vi "CAR Main.vi"(8 "error in (no error)":errorcluster) -> (0 "error out":errorcluster)   [LabVIEW 2009]
doc: "This is the main VI for the Cash Wash application. \nThis VI operates the touch-less car wash which is a car wash that relies on spray only, there are no brushes.\nSee Front Panel documentation for descriptions and tips on how to operate the car wash.\nSee Block Diagram documentation for more detailed information.\nThis VI uses a Producer Consumer (Events) Queued State Machine design pattern."
uses:
  controls/car_CarWashIndicators_cluster.ctl
  controls/car_CarWashSimulationSwitches_cluster.ctl
  controls/car_PurchaseSelection_cluster.ctl
  controls/car_ConsumerDataType_cluster.ctl
  controls/car_ConsumerCommand_enum.ctl
  modules/error/car_Error_Command_enum.ctl
  modules/car wash/car_CarWash_PurchaseSelection_enum.ctl
  modules/car wash/car_CarWash_Command_enum.ctl
panel:
  in  "Stop":bool
  in  "Simulation Switches":T1 caption="Car Wash Simulation Switches"
  out "Car Wash Indicators":T2
  in  "Purchase Selection":T3
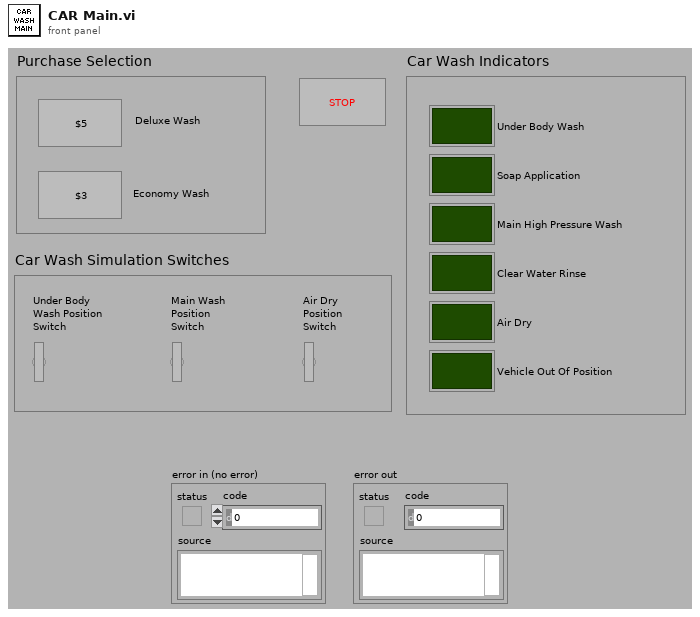
[diagram p1: front panel]
types:
  T1 = typedef "car_CarWashSimulationSwitches_cluster.ctl" = cluster{"Under Body Wash Position Switch":bool, "Main Wash Position Switch":bool, "Air Dry Position Switch":bool}
  T2 = typedef "car_CarWashIndicators_cluster.ctl" = cluster{"Under Body Wash":bool, "Soap Application":bool, "Main High Pressure Wash":bool, "Clear Water Rinse":bool, "Air Dry":bool, "Vehicle Out Of Position":bool}
  T3 = typedef "car_PurchaseSelection_cluster.ctl" = cluster{"Deluxe Wash":bool, "Economy Wash":bool}
  T4 = typedef "car_Error_Command_enum.ctl" = enum16{"Initialise", "Check for Error", "Report Errors"}
  T5 = typedef "car_ConsumerDataType_cluster.ctl" = cluster{"Command":T6, "Data":variant}
  T6 = typedef "car_ConsumerCommand_enum.ctl" = enum16{"Initialise", "Update Start Car Wash Display", "Start Wash", "Check Car Wash", "Car Wash Completed", "Exit"}
  T7 = typedef "car_CarWash_Command_enum.ctl" = enum16{"Initialise", "Start Car Wash", "Check Car Wash Cycle", "Next Cycle", "Shutdown"}
  T8 = enum8{"Enabled", "Disabled", "Disabled and Grayed Out"}
  T9 = typedef "car_CarWash_PurchaseSelection_enum.ctl" = enum16{"Economy", "Deluxe"}
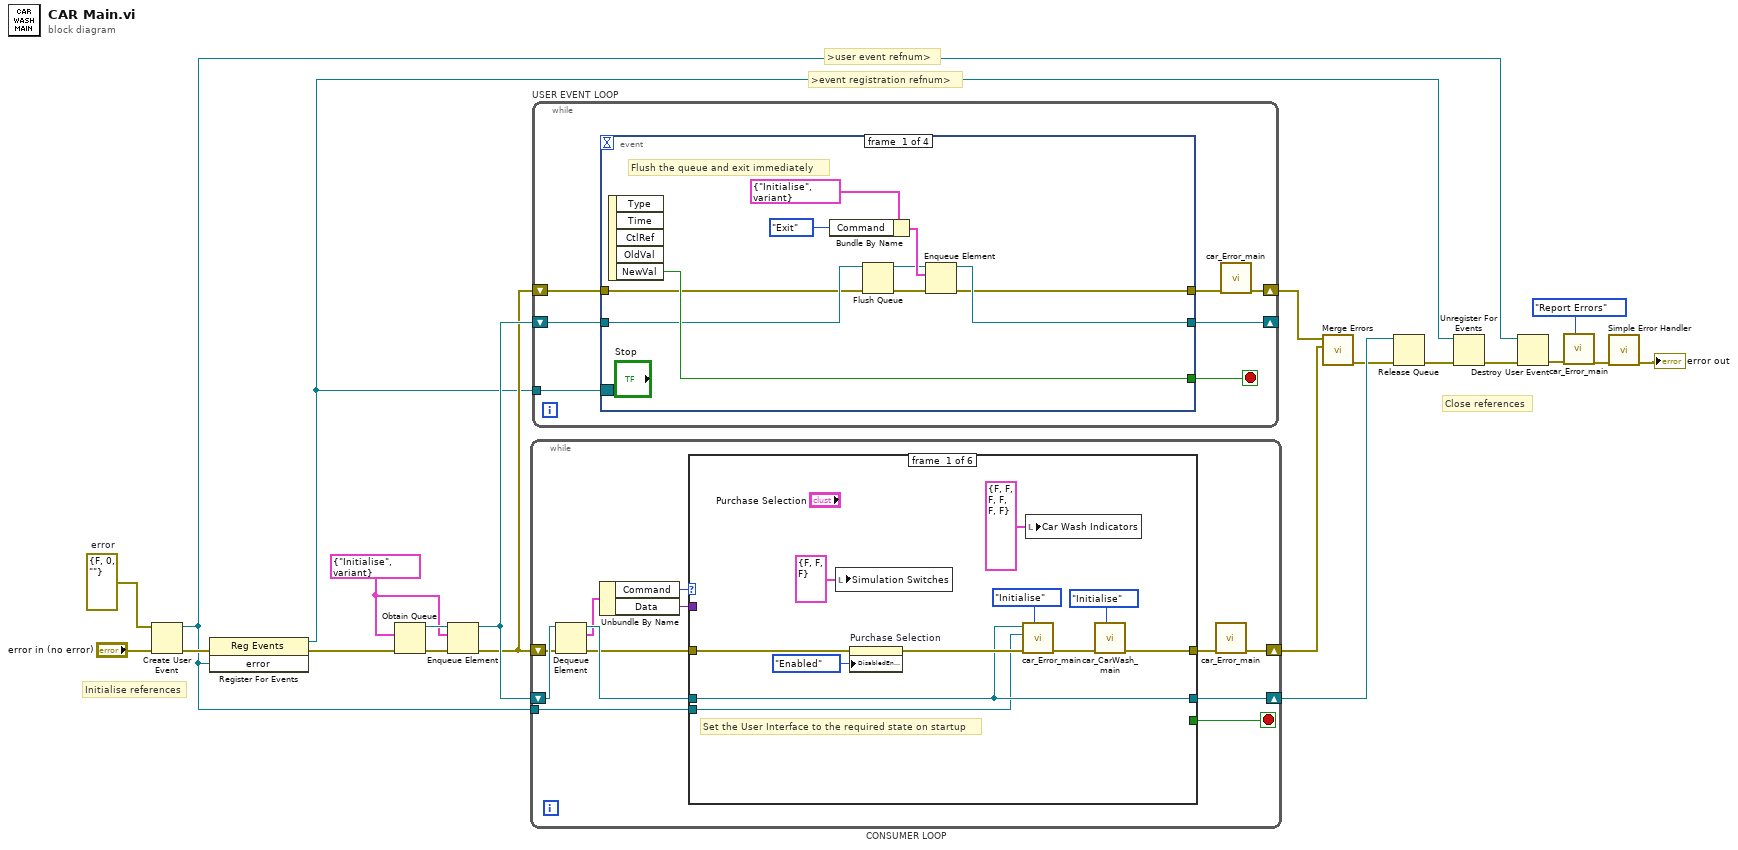
[diagram p0: block diagram]
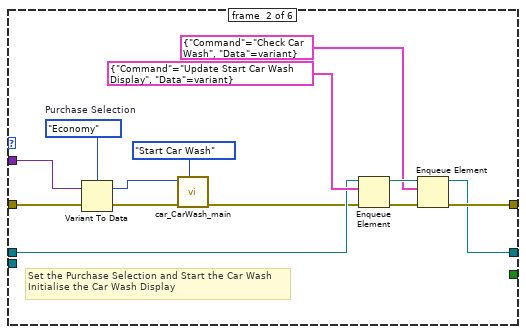
[diagram p2: hidden frame]
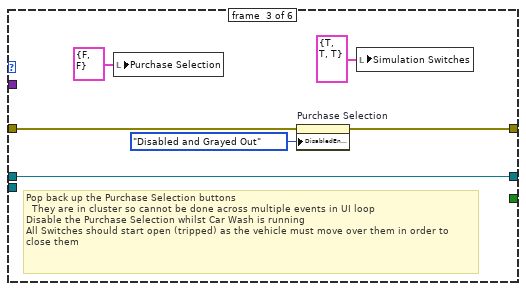
[diagram p3: hidden frame]
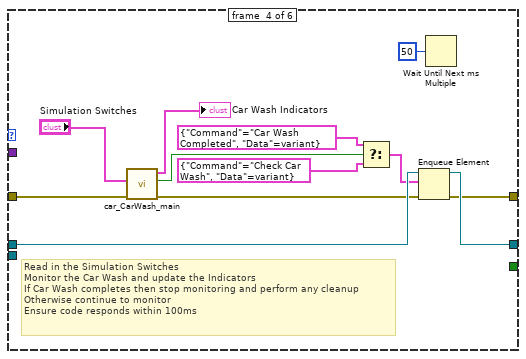
[diagram p4: hidden frame]
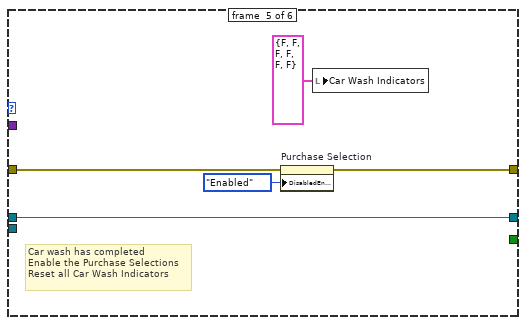
[diagram p5: hidden frame]
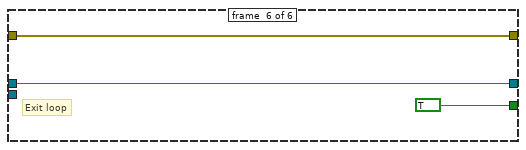
[diagram p6: hidden frame]
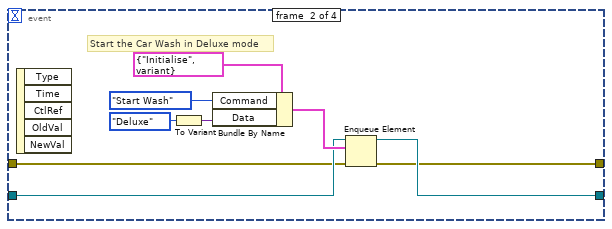
[diagram p7: hidden frame]
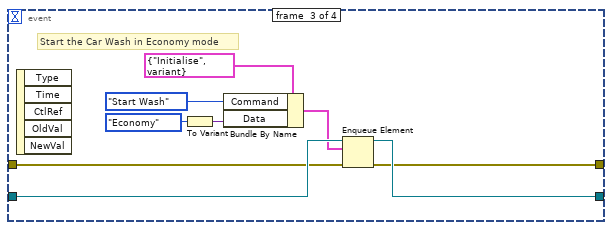
[diagram p8: hidden frame]
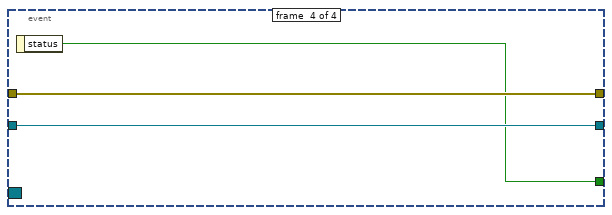
[diagram p9: hidden frame]
diagram:
  w12 = errorcluster {"status"=FALSE, "code"=0, "source"=""}  # error
  w17 = T5 {"Command"=enum."Initialise", "Data"=variant} ("Data Type")
  # "Close references"
  # ">user event refnum>"
  # ">event registration refnum>"
  # "Initialise references"
  n1 = Create User Event(user event datatype=w12, error in="error in (no error)") -> (user event=w1:refnum<user-event>, error out=w10:errorcluster)
  n2 = register-events(error in=w10, w1) -> (reference out=w7:refnum<event-registration>, error out=w9:errorcluster)  [unwired: 1 in]
  n3 = Obtain Queue(element data type=w17, error in (no error)=w9) -> (queue out=w21:refnum<queue>, error out=w20:errorcluster)  [unwired: 3 in, 1 out]
  n4 = Enqueue Element(queue=w21, element=w17, error in (no error)=w20) -> (queue out=w19:refnum<queue>, error out=w18:errorcluster)  [unwired: 1 in, 1 out]
  n5 = while "CONSUMER LOOP" {
    shift-right: [w31] -> w14
    shift-left: w19 -> [w33]
    shift-right: [w24] -> w15
    shift-left: w18 -> [w30]
    tunnel: w1 -> [w22]
    stop <- w25 stop-if-true
    n6 = Dequeue Element(queue=w33, error in (no error)=w30) -> (queue out=w32:refnum<queue>, element=w28:T5, error out=w29:errorcluster)  [unwired: 1 in, 1 out]
    n7 = Unbundle By Name(w28) -> ("Command"=w27:T6, "Data"=w26:variant)
    n8 = case shown="\"Car Wash Completed\"" w27 {
      tunnel: w32 -> [w35 w52 w64 w75 w81 w84]
      tunnel: [w35 w51 w64 w74 w81 w84] -> w31
      tunnel: [w41 w55 w60 w73 w78 w83] -> w23
      tunnel: w29 -> [w43 w58 w61 w68 w79 w83]
      tunnel: w26 -> [_ w57 _ _ _ _]
      tunnel: [_ _ _ _ _ TRUE] -> w25
      tunnel: w22 -> [w34 _ _ _ _ _]
      frame #0 {
        # "Set the User Interface to the required state on startup"
        n9 = local write "Simulation Switches"(T1 {"Under Body Wash Position Switch"=FALSE, "Main Wash Position Switch"=FALSE, "Air Dry Position Switch"=FALSE} ("Simulation Switches")) -> ()
        n10 = property on="Purchase Selection" class="Clust (strict)"(error in=w43, "DisabledEnum"=T8."Enabled" ("Disabled")) -> (error out=w38:errorcluster)  [unwired: 1 in, 1 out]
        n11 = call "car_Error_main.vi"("Command (Check for Error)"=car_Error_Command_enum."Initialise", "error in (no error)"=w38, "Error User Event"=w34, "Consumer Queue Refnum"=w35) -> ("error out"=w37:errorcluster)  [unwired: 7 in]
        n12 = local write "Car Wash Indicators"(T2 {"Under Body Wash"=FALSE, "Soap Application"=FALSE, "Main High Pressure Wash"=FALSE, "Clear Water Rinse"=FALSE, "Air Dry"=FALSE, "Vehicle Out Of Position"=FALSE} ("Car Wash Indicators")) -> ()
        n13 = call "car_CarWash_main.vi"("Command (Check Car Wash Cycle)"=car_CarWash_Command_enum."Initialise", "error in (no error)"=w37) -> ("error out"=w41:errorcluster)  [unwired: 7 in, 2 out]
      }
      frame #1 {
        w49 = car_CarWash_PurchaseSelection_enum."Economy"  # Purchase Selection
        # "Set the Purchase Selection and Start the Car Wash\nInitialise the Car Wash Display"
        n14 = Variant To Data(error in=w58, Variant=w57, type=w49) -> (error out=w48:errorcluster, data=w46:T9)
        n15 = call "car_CarWash_main.vi"("Command (Check Car Wash Cycle)"=car_CarWash_Command_enum."Start Car Wash", "error in (no error)"=w48, "Purchase Selection"=w46) -> ("error out"=w47:errorcluster)  [unwired: 6 in, 2 out]
        n16 = Enqueue Element(queue=w52, element=T5 {"Command"=enum."Update Start Car Wash Display", "Data"=variant} ("Data Type"), error in (no error)=w47) -> (queue out=w53:refnum<queue>, error out=w56:errorcluster)  [unwired: 1 in, 1 out]
        n17 = Enqueue Element(queue=w53, element=T5 {"Command"=enum."Check Car Wash", "Data"=variant} ("Data Type"), error in (no error)=w56) -> (queue out=w51:refnum<queue>, error out=w55:errorcluster)  [unwired: 1 in, 1 out]
      }
      frame #2 {
        # "Pop back up the Purchase Selection buttons \n  They are in cluster so cannot be done across multiple events in UI loop\nDisable the Purchase Selection whilst Car Wash is running\nAll Switches should start open (tripped) as the vehicle must move over them in order to close them"
        n18 = local write "Purchase Selection"(T3 {"Deluxe Wash"=FALSE, "Economy Wash"=FALSE} ("Purchase Selection")) -> ()
        n19 = property on="Purchase Selection" class="Clust (strict)"(error in=w61, "DisabledEnum"=T8."Disabled and Grayed Out" ("Disabled")) -> (error out=w60:errorcluster)  [unwired: 1 in, 1 out]
        n20 = local write "Simulation Switches"(T1 {"Under Body Wash Position Switch"=TRUE, "Main Wash Position Switch"=TRUE, "Air Dry Position Switch"=TRUE} ("Simulation Switches")) -> ()
      }
      frame #3 {
        # "Read in the Simulation Switches\nMonitor the Car Wash and update the Indicators\nIf Car Wash completes then stop monitoring and perform any cleanup\nOtherwise continue to monitor\nEnsure code responds within 100ms"
        n21 = call "car_CarWash_main.vi"("error in (no error)"=w68, "Car Wash Simulation Switches"="Simulation Switches") -> ("error out"=w67:errorcluster, "Completed Car Wash"=w65:bool, "Car Wash Indicators"=→"Car Wash Indicators":T2)  [unwired: 7 in]
        n22 = Select(t=T5 {"Command"=enum."Car Wash Completed", "Data"=variant} ("Data Type"), s=w65, f=T5 {"Command"=enum."Check Car Wash", "Data"=variant} ("Data Type")) -> (s? t:f=w70:T5)
        n23 = Enqueue Element(queue=w75, element=w70, error in (no error)=w67) -> (queue out=w74:refnum<queue>, error out=w73:errorcluster)  [unwired: 1 in, 1 out]
        n24 = Wait Until Next ms Multiple(millisecond multiple=u32 50) -> ()  [unwired: 1 out]
      }
      frame #4 {
        # "Car wash has completed\nEnable the Purchase Selections\nReset all Car Wash Indicators"
        n25 = property on="Purchase Selection" class="Clust (strict)"(error in=w79, "DisabledEnum"=T8."Enabled" ("Disabled")) -> (error out=w78:errorcluster)  [unwired: 1 in, 1 out]
        n26 = local write "Car Wash Indicators"(T2 {"Under Body Wash"=FALSE, "Soap Application"=FALSE, "Main High Pressure Wash"=FALSE, "Clear Water Rinse"=FALSE, "Air Dry"=FALSE, "Vehicle Out Of Position"=FALSE} ("Car Wash Indicators")) -> ()
      }
      frame #5 {
        # "Exit loop"
      }
    }
    n27 = call "car_Error_main.vi"("error in (no error)"=w23) -> ("error out"=w24:errorcluster)  [unwired: 10 in]
  }
  n28 = while "USER EVENT LOOP" {
    shift-right: [w88] -> _
    shift-left: w19 -> [w90]
    shift-right: [w86] -> w16
    shift-left: w18 -> [w89]
    tunnel: w7 -> [w87]
    stop <- w91 stop-if-true
    n29 = event shown="[1] \"Purchase Selection.Deluxe Wash\": Value Change" {
      selector: w87 -> [_ _ _ _]
      dyn-events: _ -> [_ _ _ _]
      timeout: _ -> [_ _ _ _]
      tunnel: [w101 _ _ w120] -> w91
      tunnel: w90 -> [w95 w104 w116 w122]
      tunnel: w89 -> [w93 w103 w115 w121]
      tunnel: [w97 w106 w114 w122] -> w88
      tunnel: [w96 w105 w113 w121] -> w85
      event #0 {
        # "Flush the queue and exit immediately"
        n30 = event-data() -> ("NewVal"=w101:bool)  [unwired: 1 in, 4 out]
        n31 = Bundle By Name(cluster=T5 {"Command"=enum."Initialise", "Data"=variant} ("Data Type"), "Command"=car_ConsumerCommand_enum."Exit") -> (w98:T5)
        n32 = Flush Queue(queue=w95, error in (no error)=w93) -> (queue out=w94:refnum<queue>, error out=w92:errorcluster)  [unwired: 1 out]
        n33 = Enqueue Element(queue=w94, element=w98, error in (no error)=w92) -> (queue out=w97:refnum<queue>, error out=w96:errorcluster)  [unwired: 1 in, 1 out]
      }
      event #1 {
        # "Start the Car Wash in Deluxe mode"
        n34 = event-data() -> ()  [unwired: 1 in, 5 out]
        n35 = To Variant(anything=car_CarWash_PurchaseSelection_enum."Deluxe" ("Purchase Selection")) -> (Variant=w108:variant)
        n36 = Bundle By Name(cluster=T5 {"Command"=enum."Initialise", "Data"=variant} ("Data Type"), "Command"=car_ConsumerCommand_enum."Start Wash", "Data"=w108) -> (w107:T5)
        n37 = Enqueue Element(queue=w104, element=w107, error in (no error)=w103) -> (queue out=w106:refnum<queue>, error out=w105:errorcluster)  [unwired: 1 in, 1 out]
      }
      event #2 {
        # "Start the Car Wash in Economy mode"
        n38 = event-data() -> ()  [unwired: 1 in, 5 out]
        n39 = To Variant(anything=car_CarWash_PurchaseSelection_enum."Economy" ("Purchase Selection")) -> (Variant=w117:variant)
        n40 = Bundle By Name(cluster=T5 {"Command"=enum."Initialise", "Data"=variant} ("Data Type"), "Command"=car_ConsumerCommand_enum."Start Wash", "Data"=w117) -> (w112:T5)
        n41 = Enqueue Element(queue=w116, element=w112, error in (no error)=w115) -> (queue out=w114:refnum<queue>, error out=w113:errorcluster)  [unwired: 1 in, 1 out]
      }
      event #3 {
        n42 = event-data() -> ("status"=w120:bool)  [unwired: 1 in]
      }
    }
    n43 = call "car_Error_main.vi"("error in (no error)"=w85) -> ("error out"=w86:errorcluster)  [unwired: 10 in]
  }
  n44 = call <vilib>:"Merge Errors.vi"("error in 2 (no error)"=w15, "error in 1 (no error)"=w16) -> ("error out"=w13:errorcluster)  [unwired: 5 in]
  n45 = Release Queue(queue=w14, error in (no error)=w13) -> (error out=w6:errorcluster)  [unwired: 1 in, 2 out]
  n46 = Unregister For Events(event registration refnum=w7, error in=w6) -> (error out=w8:errorcluster)
  n47 = Destroy User Event(user event=w1, error in=w8) -> (error out=w4:errorcluster)
  n48 = call "car_Error_main.vi"("Command (Check for Error)"=car_Error_Command_enum."Report Errors", "error in (no error)"=w4) -> ("error out"=w5:errorcluster)  [unwired: 9 in]
  n49 = call <vilib>:"Simple Error Handler.vi"("error in (no error)"=w5) -> ("error out"=→"error out":errorcluster)  [unwired: 4 in, 4 out]
